vi "Traffic Lights Simulation.vi"(4 "Stop Button":bool) -> ()   [LabVIEW 2018]
uses:
  Color states.ctl
  States.ctl
  Color times.ctl
panel:
  out "Color time 2":i32
  out "Color time 1":i32
  out "x > y?":bool
  in  "Set state":T1(ring)
  in  "Time scale":dbl
  in  "Night mode":T2=[{"yellow time"=3, "red-yellow_time"=0, "green time"=0, "red time"=0, "null time"=3}, {"yellow time"=3, "red-yellow_time"=0, "green time"=0, "red time"=0, "null time"=3}]
  in  "Traffic jam mode":T2=[{"yellow time"=10, "red-yellow_time"=5, "green time"=25, "red time"=70, "null time"=0}, {"yellow time"=10, "red-yellow_time"=5, "green time"=65, "red time"=30, "null time"=0}]
  in  "Normal mode":T2=[{"yellow time"=10, "red-yellow_time"=5, "green time"=25, "red time"=30, "null time"=0}, {"yellow time"=10, "red-yellow_time"=5, "green time"=25, "red time"=30, "null time"=0}]
  out "Current state":T3=enum."Night"
  out "Color state 2":T4
  out "Color state 1":T4
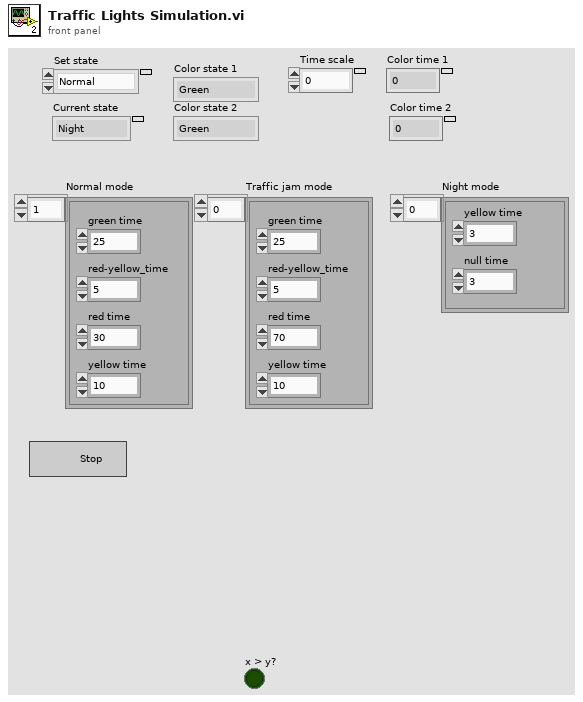
[diagram p1: front panel]
types:
  T1 = enum16{"Normal", "Night", "Traffic jam 1", "Traffic jam 2"}
  T2 = typedef "Color times.ctl" = cluster{"yellow time":i32, "red-yellow_time":i32, "green time":i32, "red time":i32, "null time":i32}[]
  T3 = typedef "States.ctl" = enum16{"Normal", "Night", "Traffic jam 1", "Traffic jam 2"}
  T4 = typedef "Color states.ctl" = enum16{"Green", "Red-Yellow", "Yellow", "Red", "Null"}
  T5 = cluster{"fractional second":dbl, "second":i32, "minute":i32, "hour":i32, "day of month":i32, "month":i32, "year":i32, "day of week":i32, "day of year":i32, "DST":i32}
  T6 = cluster{"yellow time":i32, "red-yellow_time":i32, "green time":i32, "red time":i32, "null time":i32}
  T7 = cluster{"yellow time":i32, "red-yellow_time":i32, "green time":i32, "red time":i32, "null time":i32}[]
  T8 = typedef "LVDateTimeRec.ctl" = cluster{"fractional second":dbl, "second":i32, "minute":i32, "hour":i32, "day of month":i32, "month":i32, "year":i32, "day of week":i32, "day of year":i32, "DST":i32}
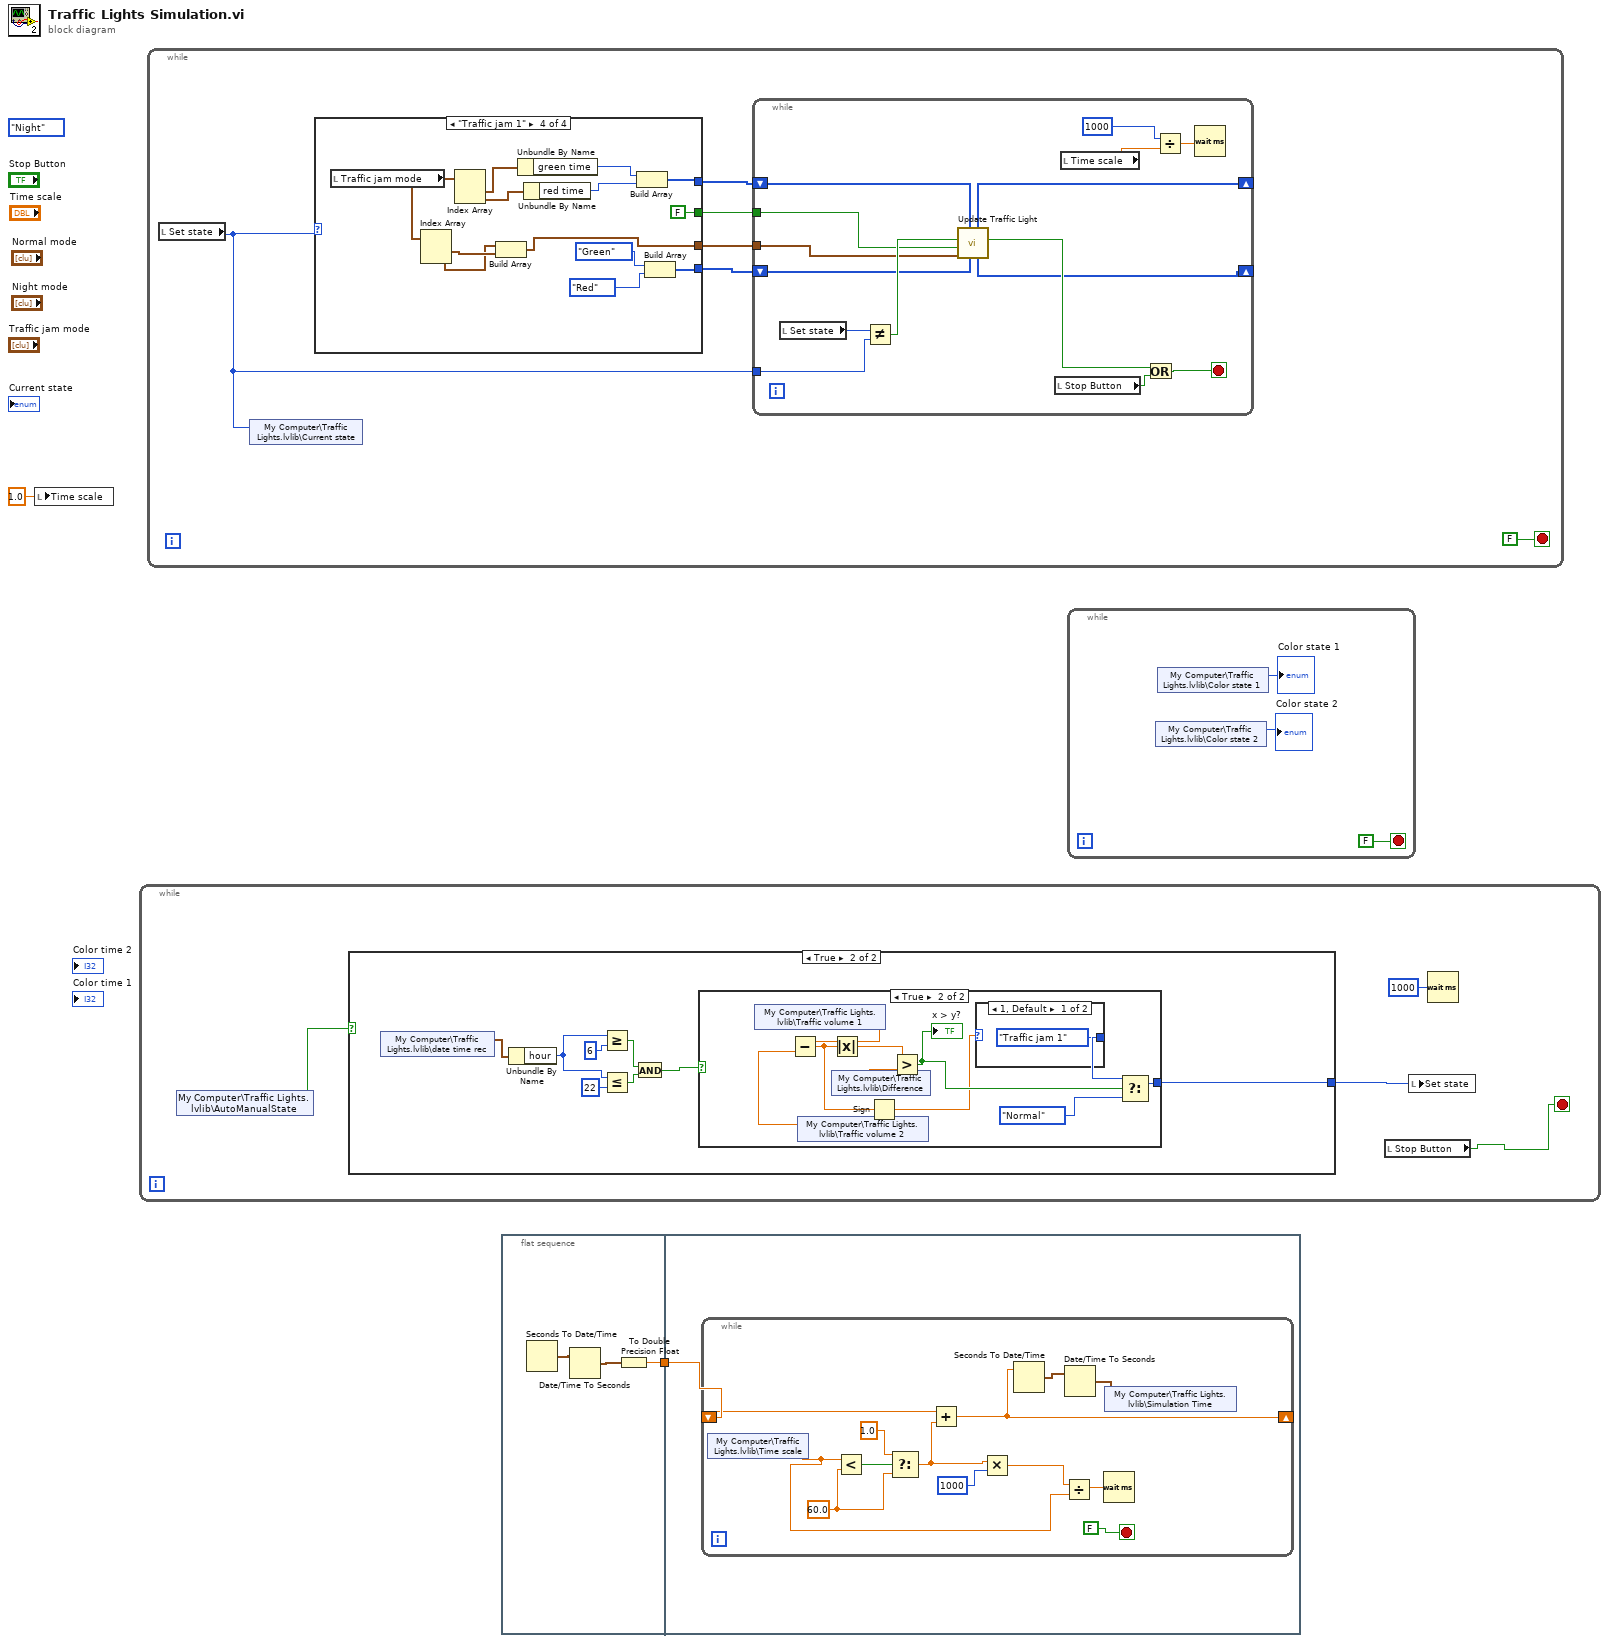
[diagram p0: block diagram]
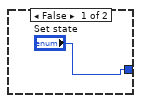
[diagram p2: hidden frame]
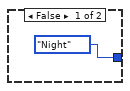
[diagram p3: hidden frame]
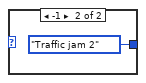
[diagram p4: hidden frame]
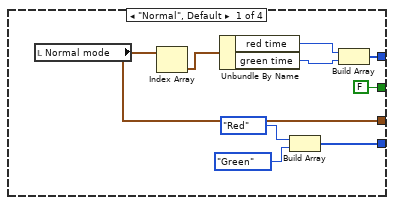
[diagram p5: hidden frame]
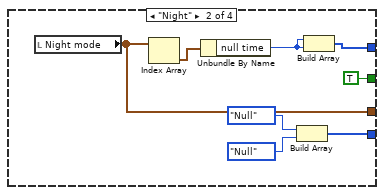
[diagram p6: hidden frame]
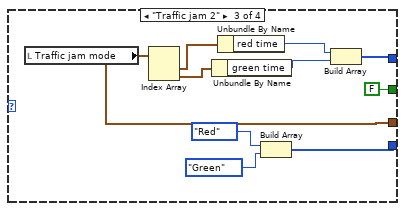
[diagram p7: hidden frame]
diagram:
  (unwired) States."Night"
  n1 = local write "Time scale"(1.0 ("Time scale")) -> ()
  n2 = while {
    stop <- w3 stop-if-true
    n3 = shared-variable "My Computer\\Traffic Lights.lvlib\\AutoManualState"() -> (w5:bool)  [unwired: 1 in, 1 out]
    n4 = case shown="True" w5 {
      tunnel: ["Set state" w10] -> w4
      frame False {
      }
      frame True {
        n5 = shared-variable "My Computer\\Traffic Lights.lvlib\\date time rec"() -> (w9:T5)  [unwired: 1 in, 1 out]
        n6 = Unbundle By Name(w9) -> ("hour"=w8:i32)
        n7 = Greater Or Equal?(x=w8, y=6 ("x")) -> (x >= y?=w15:bool)
        n8 = Less Or Equal?(x=w8, y=22) -> (x <= y?=w13:bool)
        n9 = And(x=w15, y=w13) -> (x .and. y?=w12:bool)
        n10 = case shown="True" w12 {
          tunnel: [T1."Night" ("Set state") w19] -> w10
          frame False {
          }
          frame True {
            n11 = shared-variable "My Computer\\Traffic Lights.lvlib\\Traffic volume 1"() -> (w26:dbl)  [unwired: 1 in, 1 out]
            n12 = shared-variable "My Computer\\Traffic Lights.lvlib\\Traffic volume 2"() -> (w25:dbl)  [unwired: 1 in, 1 out]
            n13 = Subtract(x=w26, y=w25) -> (x-y=w21:dbl)
            n14 = Absolute Value(x=w21) -> (abs(x)=w24:dbl)
            n15 = shared-variable "My Computer\\Traffic Lights.lvlib\\Difference"() -> (w23:dbl)  [unwired: 1 in, 1 out]
            n16 = Sign(1:w21) -> (0:w18:dbl)
            n17 = Greater?(x=w24, y=w23) -> (0:w22:bool)
            "x > y?" <- w22
            n18 = case shown="1, Default" w18 {
              tunnel: [T1."Traffic jam 1" ("Set state") T1."Traffic jam 2" ("Set state")] -> w17
              frame 1, Default {
              }
              frame -1 {
              }
            }
            n19 = Select(t=w17, s=w22, f=T1."Normal" ("Set state")) -> (s? t:f=w19:T1)
          }
        }
      }
    }
    n20 = local read "Stop Button"() -> (w3:bool)
    n21 = local write "Set state"(w4) -> ()
    n22 = Wait (ms)(milliseconds to wait=u32 1000) -> ()  [unwired: 1 out]
  }
  n23 = while {
    stop <- FALSE stop-if-true
    n24 = local read "Set state"() -> (w29:T1)
    n25 = shared-variable "My Computer\\Traffic Lights.lvlib\\Current state"(w29) -> ()  [unwired: 1 in, 1 out]
    n26 = case shown="\"Traffic jam 1\"" w29 {
      tunnel: [w38 w49 w56 w70] -> w33
      tunnel: [w39 w47 w55 w69] -> w32
      tunnel: [w37 w46 w57 w62] -> w31
      tunnel: [FALSE ("Blinking") TRUE ("Blinking") FALSE ("Blinking") FALSE ("Blinking")] -> w30
      frame "Normal", Default {
        n27 = local read "Normal mode"() -> (w37:T2)
        n28 = Index Array(array=w37) -> (element=w42:T6)  [unwired: 1 in]
        n29 = Unbundle By Name(w42) -> ("red time"=w43:i32, "green time"=w35:i32)
        n30 = Build Array(Color_states."Red", Color_states."Green") -> (w38:T4[])
        n31 = Build Array(w43, w35) -> (w39:i32[])
      }
      frame "Night" {
        n32 = local read "Night mode"() -> (w46:T2)
        n33 = Index Array(array=w46) -> (element=w48:T6)  [unwired: 1 in]
        n34 = Unbundle By Name(w48) -> ("null time"=w44:i32)
        n35 = Build Array(Color_states."Null", Color_states."Null") -> (w49:T4[])
        n36 = Build Array(w44, w44) -> (w47:i32[])
      }
      frame "Traffic jam 2" {
        n37 = local read "Traffic jam mode"() -> (w57:T2)
        n38 = Index Array(array=w57) -> (element #1=w61:T6, element #2=w54:T6)  [unwired: 2 in]
        n39 = Unbundle By Name(w54) -> ("green time"=w53:i32)
        n40 = Unbundle By Name(w61) -> ("red time"=w60:i32)
        n41 = Build Array(Color_states."Red", Color_states."Green") -> (w56:T4[])
        n42 = Build Array(w60, w53) -> (w55:i32[])
      }
      frame "Traffic jam 1" {
        n43 = local read "Traffic jam mode"() -> (w65:T2)
        n44 = Index Array(array=w65) -> (element #1=w64:T6, element #2=w63:T6)  [unwired: 2 in]
        n45 = Index Array(array=w65) -> (element #1=w74:T6, element #2=w68:T6)  [unwired: 2 in]
        n46 = Build Array(w63, w64) -> (w62:T7)
        n47 = Unbundle By Name(w74) -> ("green time"=w73:i32)
        n48 = Unbundle By Name(w68) -> ("red time"=w67:i32)
        n49 = Build Array(w73, w67) -> (w69:i32[])
        n50 = Build Array(Color_states."Green", Color_states."Red") -> (w70:T4[])
      }
    }
    n51 = while {
      shift-right: [w76] -> _
      shift-left: w33 -> [w78]
      tunnel: w29 -> [w81]
      shift-right: [w75] -> _
      shift-left: w32 -> [w77]
      tunnel: w31 -> [w79]
      tunnel: w30 -> [w82]
      stop <- w89 stop-if-true
      n52 = local read "Set state"() -> (w80:T1)
      n53 = Not Equal?(x=w80, y=w81) -> (x != y?=w85:bool)
      n54 = call "Update Traffic Light.vi"("Color state in"=w78, "Time in"=w77, "Color times"=w79, "Blinking"=w82, "Sync in"=w85) -> ("Sync out"=w83:bool, "Color state out"=w76:T4[], "Time out"=w75:i32[])  [unwired: 4 in]
      n55 = local read "Stop Button"() -> (w84:bool)
      n56 = local read "Time scale"() -> (w87:dbl)
      n57 = Or(x=w83, y=w84) -> (x .or. y?=w89:bool)
      n58 = Divide(x=u32 1000 ("milliseconds to wait"), y=w87) -> (x/y=w88:dbl)
      n59 = Wait (ms)(milliseconds to wait=w88) -> ()  [unwired: 1 out]
    }
  }
  n60 = flat-sequence {
    tunnel: [w90] -> w1
    tunnel: w1 -> [w93]
    frame #0 {
      n61 = Seconds To Date/Time() -> (date time rec=w92:T8)  [unwired: 2 in]
      n62 = Date/Time To Seconds(2:w92) -> (0:w91:timestamp)  [unwired: 1 in]
      n63 = To Double Precision Float(number=w91) -> (double precision float=w90:dbl)
    }
    frame #1 {
      n64 = while {
        shift-right: [w104] -> _
        shift-left: w93 -> [w105]
        stop <- FALSE stop-if-true
        w99 = 60.0 ("f")
        n65 = shared-variable "My Computer\\Traffic Lights.lvlib\\Time scale"() -> (w100:dbl)  [unwired: 1 in, 1 out]
        n66 = Less?(x=w100, y=w99) -> (x < y?=w101:bool)
        n67 = Select(t=1.0, s=w101, f=w99) -> (s? t:f=w97:dbl)
        n68 = Add(x=w105, y=w97) -> (x+y=w104:dbl)
        n69 = Multiply(x=w97, y=u32 1000 ("milliseconds to wait")) -> (x*y=w96:dbl)
        n70 = Seconds To Date/Time(time stamp (now)=w104) -> (date time rec=w95:T8)  [unwired: 1 in]
        n71 = Divide(x=w96, y=w100) -> (x/y=w103:dbl)
        n72 = Date/Time To Seconds(2:w95) -> (0:w94:timestamp)  [unwired: 1 in]
        n73 = Wait (ms)(milliseconds to wait=w103) -> ()  [unwired: 1 out]
        n74 = shared-variable "My Computer\\Traffic Lights.lvlib\\Simulation Time"(w94) -> ()  [unwired: 1 in, 1 out]
      }
    }
  }
  n75 = while {
    stop <- FALSE stop-if-true
    n76 = shared-variable "My Computer\\Traffic Lights.lvlib\\Color state 2"() -> (→"Color state 2":T4)  [unwired: 1 in, 1 out]
    n77 = shared-variable "My Computer\\Traffic Lights.lvlib\\Color state 1"() -> (→"Color state 1":T4)  [unwired: 1 in, 1 out]
  }
